vi "Initialize Hardware References.vi"(8 "error in (no error)":errorcluster, 11 "Hardware Resources in":T1={"DAQmx Task"="", "Counter(s)"="Dev2/ctr0", "samples per readout"=0}) -> (0 "error out":errorcluster, 3 "Hardware Resources out":T1={"DAQmx Task"="", "Counter(s)"="Dev2/ctr0", "samples per readout"=0})   [LabVIEW 2013, in "Acquisition.lvlib"]
doc: "Initialize the hardware references."
uses:
  Acquisition.lvlib
  Hardware Configuration.ctl
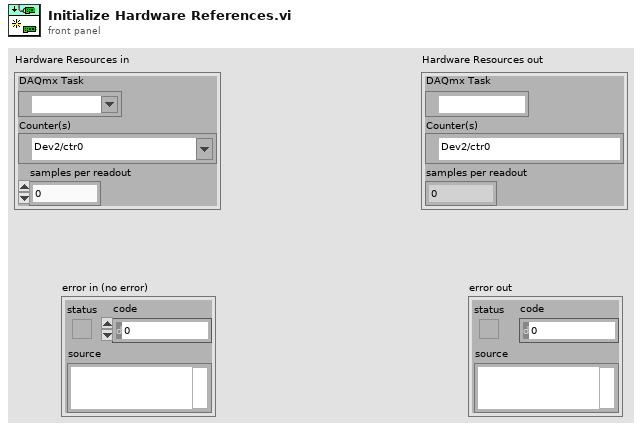
[diagram p1: front panel]
types:
  T1 = typedef "Acquisition.lvlib/Hardware Configuration.ctl" = cluster{"DAQmx Task":refnum<k21>, "Counter(s)":tag, "samples per readout":i32}
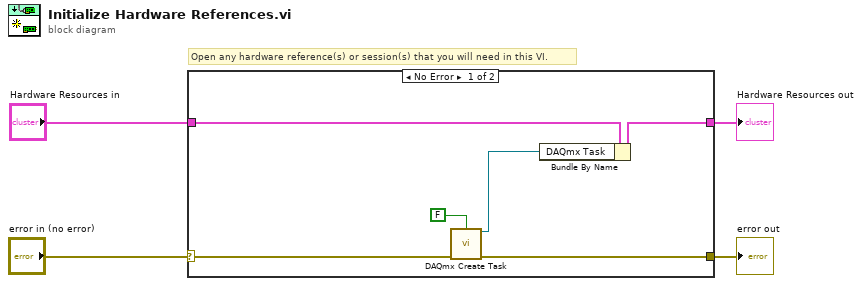
[diagram p0: block diagram]
diagram:
  # "Open any hardware reference(s) or session(s) that you will need in this VI."
  n1 = case shown="No Error" "error in (no error)" {
    selector: "error in (no error)" -> [w7 w11]
    tunnel: [w5 w11] -> w3
    tunnel: "Hardware Resources in" -> [w9 w12]
    tunnel: [w10 w12] -> w1
    frame No Error {
      n2 = call <vilib>:"DAQmx Create Task.vi"("auto cleanup"=FALSE, "error in"=w7) -> ("task out"=w6:refnum<k21>, "error out"=w5:errorcluster)  [unwired: 12 in]
      n3 = Bundle By Name(cluster=w9, "DAQmx Task"=w6) -> (w10:T1)
    }
    frame Error {
    }
  }
  "Hardware Resources out" <- w1
  "error out" <- w3
